vi "Draw.vi"(8 "error in (no error)":errorcluster, 10 "Picture in":picture, 11 "Line in":refnum<class "Line.lvclass">) -> (0 "error out":errorcluster, 2 "Picture out":picture, 3 "Line out":refnum<class "Line.lvclass">)   [LabVIEW 2015, in "Line.lvclass"]
uses:
  Line.lvclass
  Interfaces/Shape/Shape.lvclass/Shape.ctl
  Interfaces/Shape/Shape.lvclass
panel:
  # "NOTICE -- YOU MUST LEAVE THIS NOTICE IN PLACE.\n\nCopyright (c) 2017, LIANG LIU Shawn.Liu.cn@gmail.com\nAll rights reserved.\n\nRedistribution and use in source and binary forms, with or without modification, are permitted provided that the following conditions are met:\n-Redistributions of source code must retain the above copyright notice, this list of conditions and the following disclaimer.\n-Redistributions in binary form must reproduce the above copyright notice, this list of conditions and the following disclaimer in the documentation and/or other materials provided with the distribution.\n-Neither the name of the eLp nor the names of its contributors may be used to endorse or promote products derived from this software without specific prior written permission.\n\nTHIS SOFTWARE IS PROVIDED BY THE COPYRIGHT HOLDERS AND CONTRIBUTORS \"AS IS\" AND ANY EXPRESS OR IMPLIED WARRANTIES, INCLUDING, BUT NOT LIMITED TO, THE IMPLIED WARRANTIES OF MERCHANTABILITY AND FITNESS FOR A PARTICULAR PURPOSE ARE DISCLAIMED. IN NO EVENT SHALL THE COPYRIGHT HOLDER OR CONTRIBUTORS BE LIABLE FOR ANY DIRECT, INDIRECT, INCIDENTAL, SPECIAL, EXEMPLARY, OR CONSEQUENTIAL DAMAGES (INCLUDING, BUT NOT LIMITED TO, PROCUREMENT OF SUBSTITUTE GOODS OR SERVICES; LOSS OF USE, DATA, OR PROFITS; OR BUSINESS INTERRUPTION) HOWEVER CAUSED AND ON ANY THEORY OF LIABILITY, WHETHER IN CONTRACT, STRICT LIABILITY, OR TORT (INCLUDING NEGLIGENCE OR OTHERWISE) ARISING IN ANY WAY OUT OF THE USE OF THIS SOFTWARE, EVEN IF ADVISED OF THE POSSIBILITY OF SUCH DAMAGE."
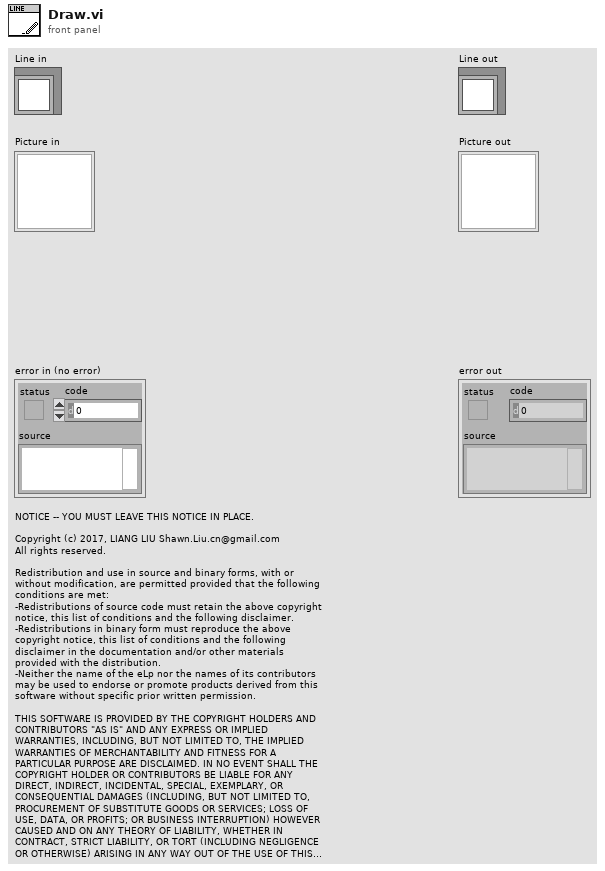
[diagram p1: front panel]
types:
  T1 = cluster{"Width":u16, "Style":enum32{"Solid", "Dash", "Dot", "DashDot", "DashDotDot"}}
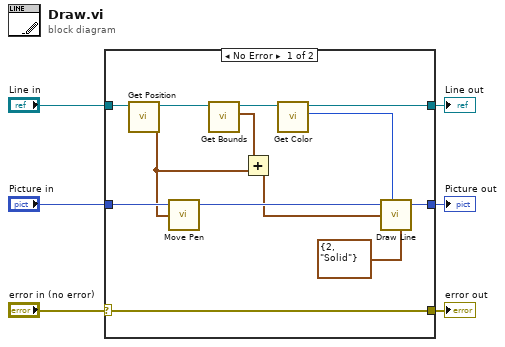
[diagram p0: block diagram]
diagram:
  n1 = case shown="No Error" "error in (no error)" {
    selector: "error in (no error)" -> [w16 w22]
    tunnel: "Picture in" -> [w19 w20]
    tunnel: [w18 w21] -> w5
    tunnel: [w17 w20] -> w4
    tunnel: "Line in" -> [w7 w21]
    tunnel: [w16 w22] -> w1
    frame No Error {
      n2 = call "Get Position.vi"("Shape in"=w7) -> ("Position"=w10:cluster{"Left":i32, "Top":i32}, "Shape out"=w9:refnum<class "Line.lvclass">)  [unwired: 9 in]
      n3 = call <vilib>:"Move Pen.vi"("new position"=w10, "picture"=w19) -> ("new picture"=w14:picture)  [unwired: 3 in]
      n4 = call "Get Bounds.vi"("Shape in"=w9) -> ("Bounds"=w11:cluster{"Width":u32, "Height":u32}, "Shape out"=w8:refnum<class "Line.lvclass">)  [unwired: 9 in]
      n5 = Add(x=w11, y=w10) -> (x+y=w13:cluster{u32, u32})
      n6 = call "Get Color.vi"("Shape in"=w8) -> ("Color"=w15:u32, "Shape out"=w18:refnum<class "Line.lvclass">)  [unwired: 9 in]
      n7 = call <vilib>:"Draw Line.vi"("picture"=w14, "end point"=w13, "color(black)"=w15, "pen"=T1 {"Width"=2, "Style"=enum."Solid"}) -> ("new picture"=w17:picture)  [unwired: 5 in]
    }
    frame Error {
    }
  }
  "error out" <- w1
  "Line out" <- w5
  "Picture out" <- w4
